vi "MultiChannelType_1D-Array-3DPoints-I32.vi"(9 "error in":errorcluster, 11 "Array in":T1[](array[typedef])) -> (1 "error out":errorcluster, 2 "MultiChannelType":T1, 3 "Array out":T1[](array[typedef]))   [LabVIEW 2020, in "OpenLvVision_OpenCv.lvlib"]
uses:
  <vilib>/Utility/error.llb/Error Cluster From Error Code.vi
  <vilib>/ErrorRing/Error Ring.xnode
  OpenLvVision_OpenCv.lvlib
  TypeDef/Point/3D_PointI32.ctl
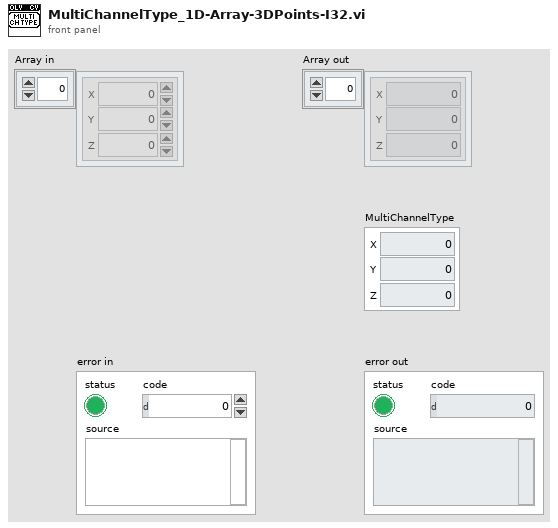
[diagram p1: front panel]
types:
  T1 = typedef "OpenLvVision_OpenCv.lvlib/3D_PointI32.ctl" = cluster{"X":i32, "Y":i32, "Z":i32}
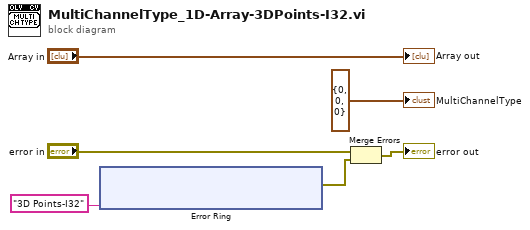
[diagram p0: block diagram]
diagram:
  n1 = xnode "Error Ring"("parameter 0"="3D Points-I32") -> ("error out"=w2:errorcluster)
  n2 = Merge Errors("error in", w2) -> (→"error out":errorcluster)
  "Array out" <- "Array in"
  "MultiChannelType" <- T1 {"X"=0, "Y"=0, "Z"=0} ("MultiChannelType")
